vi "EngineTagsUI.vi"() -> ()   [LabVIEW 2013, in "PL Framework Configuration Tool.lvlib" / "Engine Mappings.lvclass"]
uses:
  Engine Mappings.lvclass
  <vilib>/CEF_TreeControl/Node/NodeRef.ctl
  <vilib>/CEF_TreeControl/Node/NISE_CEF_Node.lvclass
  <vilib>/NI/AMC/Message Queue.ctl
  <vilib>/NI/AMC/Message.ctl
  <vilib>/NI/Tools/Keyed Array/KeyedArray.ctl
  <vilib>/CEF_TreeControl/Node/UserEventRef.ctl
  <vilib>/CEF_TreeControl/Controls/EventCluster.ctl
  <vilib>/NI/Tag Bus Module Framework/root configuration/TBM configuration.lvclass/TBM configuration.ctl
  <vilib>/NI/Tag Bus/tag/tag descriptor.lvclass/tag descriptor.ctl
  Engine Parent/read engine configuration.vi
  <vilib>/NI/Tag Bus Module Framework/root configuration/create GUID.vi
  Engine Parent/write engine configuration.vi
  <vilib>/NI/Module Execution Interface/Engine Configuration/engine configuration.lvclass
  <vilib>/NI/Tag Bus Module Framework/root configuration/TBM configuration.lvclass
  Engine Parent/Engine Parent Editor Node.lvclass
  <vilib>/CEF_TreeControl/NISE_CEF_TreeControl.lvlib
  <vilib>/NI/Tag Bus/tag/tag descriptor.lvclass
  <vilib>/NI/Tools/Keyed Array/Tools_KeyedArray.lvlib
  <vilib>/NI/AMC/AMC.lvlib
panel:
  in  "channels":i32(listbox)
  in  "main queue":T1
  in  "node ref":T2
  in  "Tags":i32(listbox)
  in  "user event":T3
  in  "unmap":bool
  in  "map":bool
  in  "Mappings":i32(listbox)
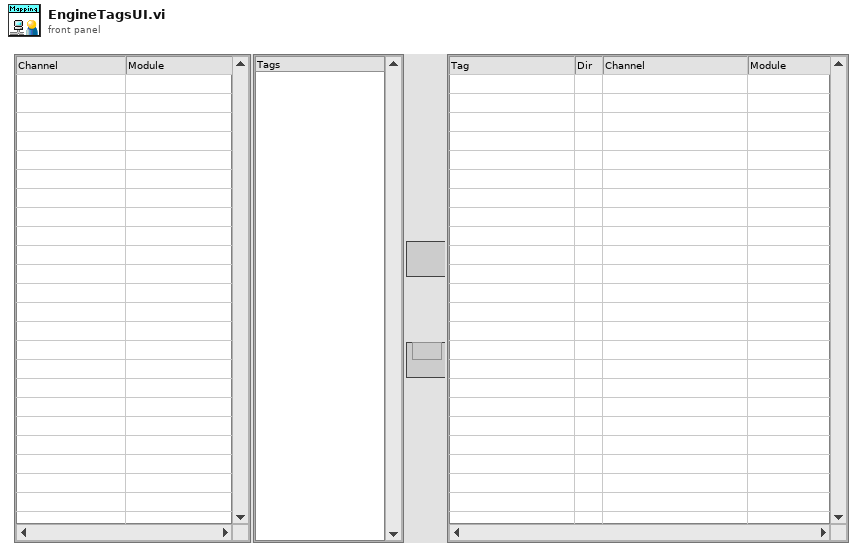
[diagram p1: front panel]
types:
  T1 = typedef "AMC.lvlib/Message Queue.ctl" = refnum<queue>
  T2 = typedef "NISE_CEF_Node.lvclass/NodeRef.ctl" = refnum<data-value>
  T3 = typedef "NISE_CEF_Node.lvclass/UserEventRef.ctl" = refnum<user-event>
  T4 = typedef "NISE_CEF_TreeControl.lvlib/EventCluster.ctl" = cluster{"command":string, "data":string}
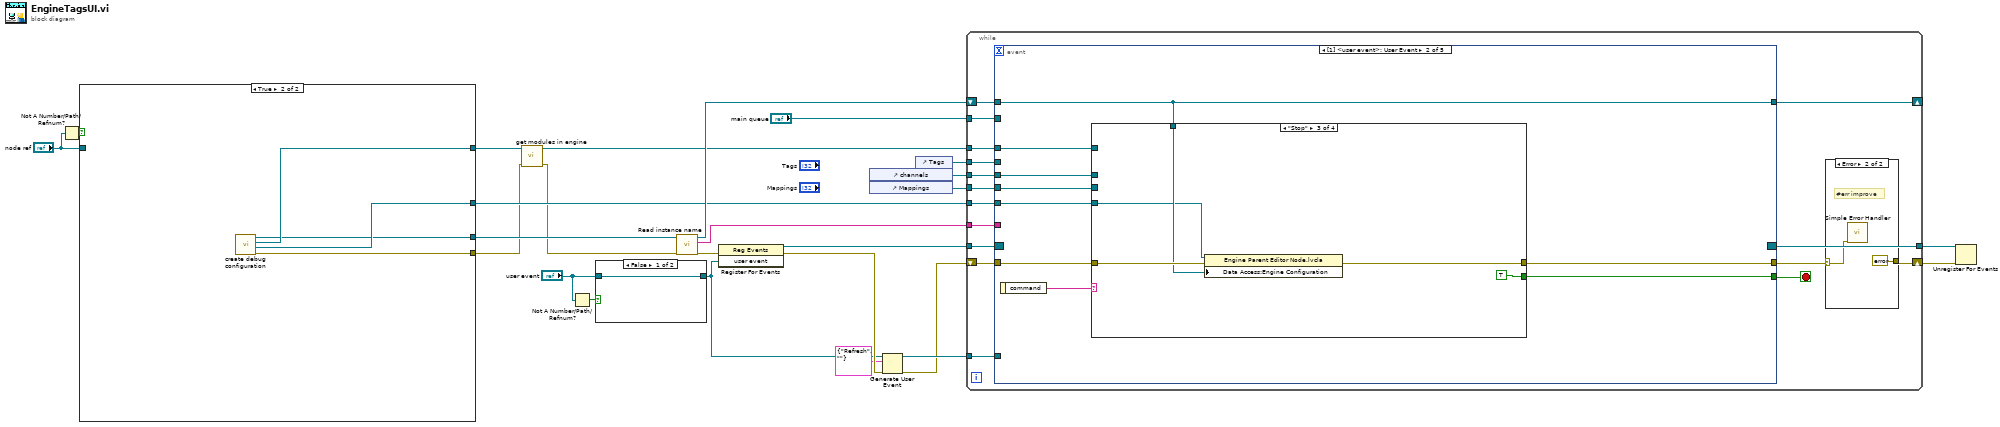
[diagram p0: block diagram]
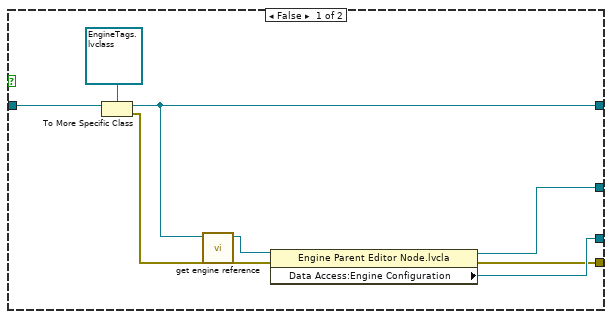
[diagram p2: hidden frame]
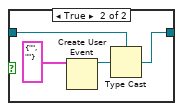
[diagram p3: hidden frame]
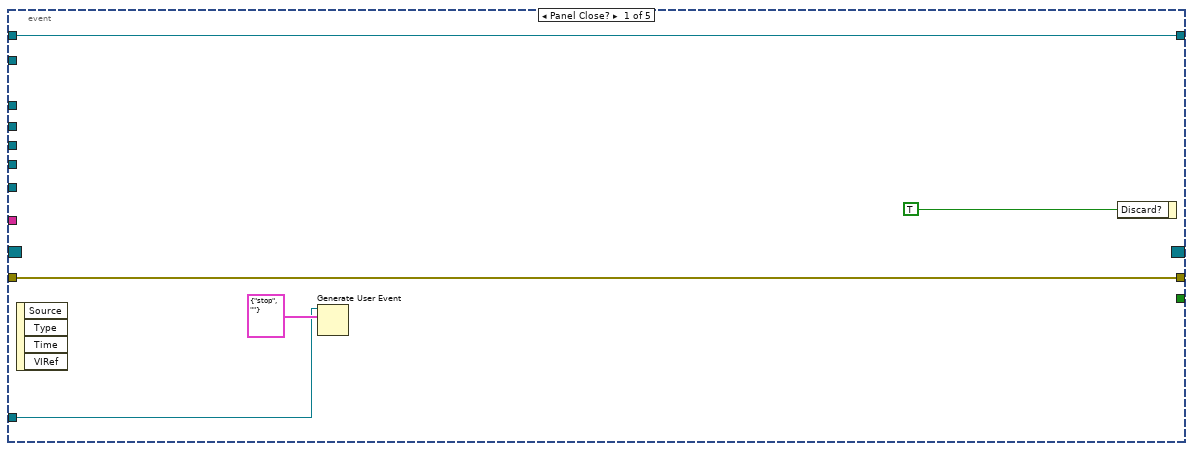
[diagram p5: hidden frame]
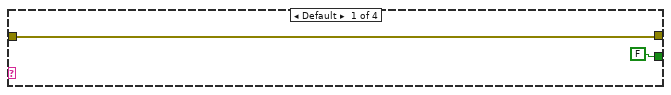
[diagram p6: hidden frame]
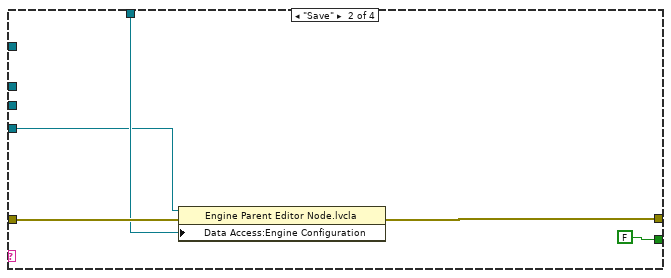
[diagram p7: hidden frame]
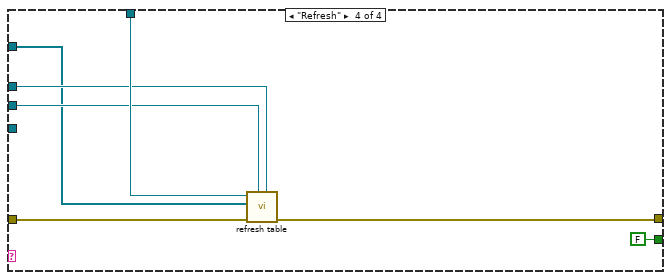
[diagram p8: hidden frame]
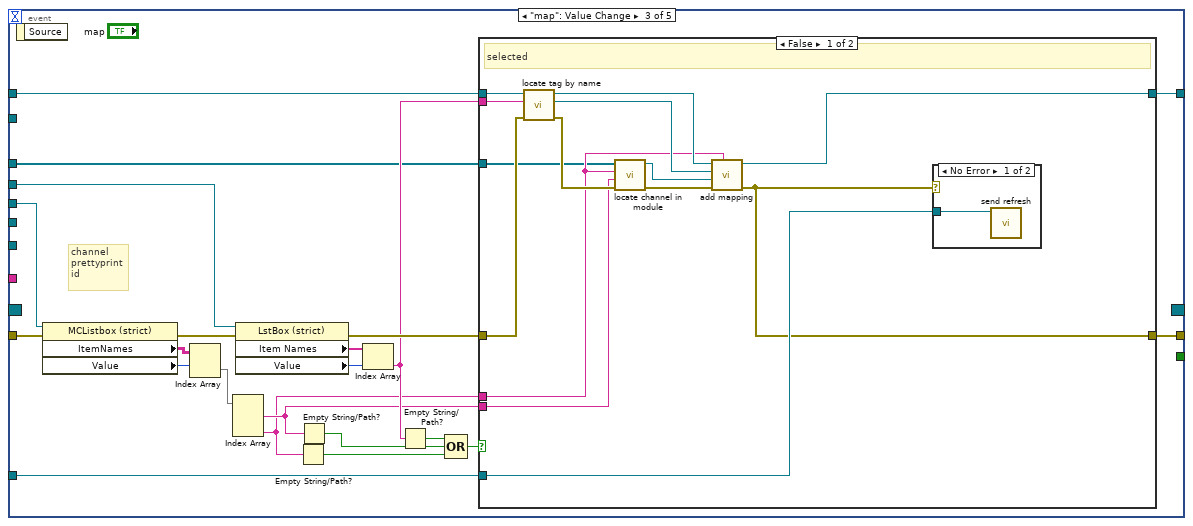
[diagram p9: hidden frame]
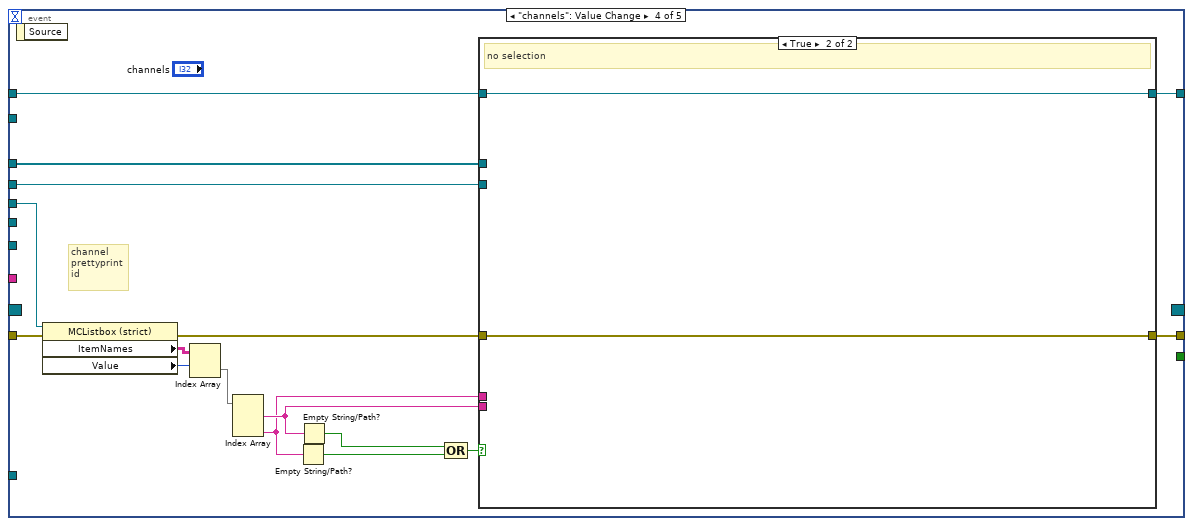
[diagram p12: hidden frame]
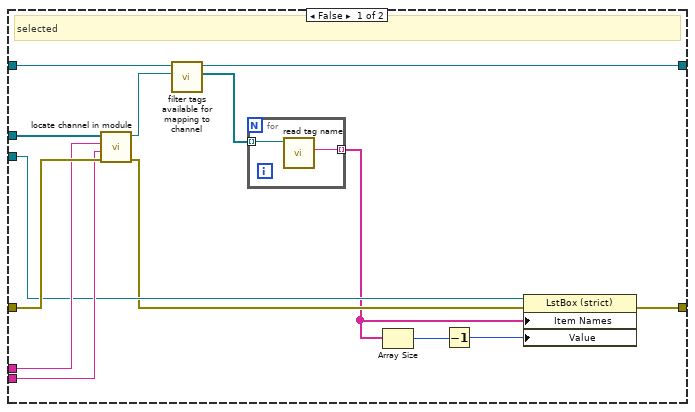
[diagram p13: hidden frame]
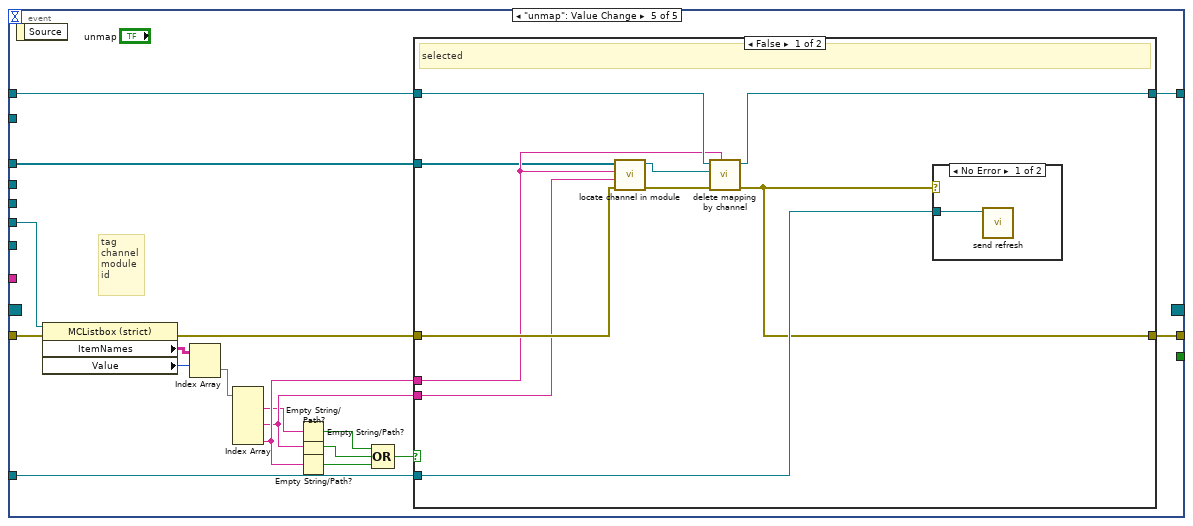
[diagram p14: hidden frame]
diagram:
  n1 = Not A Number/Path/Refnum?(number/path/refnum="node ref") -> (NaN/Path/Refnum?=w12:bool)
  n2 = case shown="True" w12 {
    tunnel: [w31 w37] -> w4
    tunnel: [w29 w36] -> w19
    tunnel: [w28 w35] -> w2
    tunnel: [w27 w38] -> w16
    tunnel: "node ref" -> [w26 _]
    frame False {
      n3 = To More Specific Class(target class=refnum<data-value> refnum ("data value reference"), reference=w26) -> (specific class reference=w31:refnum<data-value>, error out=w33:errorcluster)  [unwired: 1 in]
      n4 = call "get engine reference.vi"("error in"=w33, "engine mappings"=w31) -> ("error out"=w32:errorcluster, "engine reference"=w30:refnum<data-value>)  [unwired: 8 in]
      n5 = property class="Engine Parent Editor Node.lvcla"(reference=w30, error in=w32) -> (reference out=w27:refnum<data-value>, error out=w28:errorcluster, "Data Access:Engine Configuration"=w29:refnum<class "engine configuration.lvclass">)
    }
    frame True {
      n6 = call "create debug configuration.vi"() -> ("error out"=w35:errorcluster, "engine dvr"=w38:refnum<data-value>, "mapping dvr"=w37:refnum<data-value>, "engine configuration out"=w36:refnum<class "engine configuration.lvclass">)  [unwired: 8 in]
    }
  }
  n7 = call "get modules in engine.vi"("error in"=w2, "engine mapping"=w4) -> ("error out"=w1:errorcluster, "Modules Configurations"=w3:refnum<class "TBM module configuration.lvclass">[])  [unwired: 8 in]
  n8 = Not A Number/Path/Refnum?(number/path/refnum="user event") -> (NaN/Path/Refnum?=w14:bool)
  n9 = case shown="False" w14 {
    tunnel: [w39 w40] -> w11
    tunnel: "user event" -> [w39 w41]
    frame False {
    }
    frame True {
      n10 = Create User Event(user event datatype=T4 {"command"="", "data"=""} ("event data")) -> (user event=w42:refnum<user-event>)  [unwired: 1 in, 1 out]
      n11 = Type Cast(type=w41, x=w42) -> (*(type *) &x=w40:T3)
    }
  }
  n12 = call <vilib>:"Read instance name.vi"("error in"=w1, "configuration in"=w19) -> ("error out"=w17:errorcluster, "instance id"=w18:string, "configuration out"=w20:refnum<class "engine configuration.lvclass">)  [unwired: 7 in]
  n13 = register-events(error in=w17, w11) -> (reference out=w24:refnum<event-registration>, error out=w21:errorcluster)  [unwired: 1 in]
  n14 = control-ref of="channels"() -> (w6:refnum<vi>)
  n15 = control-ref of="Mappings"() -> (w5:refnum<vi>)
  n16 = Generate User Event(user event=w11, event data cluster=T4 {"command"="Refresh", "data"=""} ("event data"), error in=w21) -> (user event out=w10:T3, error out=w9:errorcluster)  [unwired: 1 in]
  n17 = control-ref of="Tags"() -> (w7:refnum<vi>)
  n18 = while {
    tunnel: "main queue" -> [w59]
    tunnel: w24 -> [w58]
    tunnel: [w57] -> w23
    shift-right: [w55] -> _
    shift-left: w20 -> [w50]
    shift-right: [w54] -> w22
    shift-left: w9 -> [w53]
    tunnel: w18 -> [w52]
    tunnel: w16 -> [w51]
    tunnel: w10 -> [w48]
    tunnel: w7 -> [w47]
    tunnel: w6 -> [w46]
    tunnel: w5 -> [w45]
    tunnel: w3 -> [w44]
    stop <- w56 stop-if-true
    n19 = event shown="[1] <user event>: User Event" {
      selector: w58 -> [_ _ _ _ _]
      dyn-events: [_ _ _ _ _] -> w57
      timeout: _ -> [_ _ _ _ _]
      tunnel: w59 -> [_ _ _ _ _]
      tunnel: [_ w72 _ _ _] -> w56
      tunnel: w50 -> [w67 w74 w103 w140 w178]
      tunnel: [w67 w74 w104 w141 w179] -> w55
      tunnel: w53 -> [w66 w76 w117 w150 w186]
      tunnel: [w66 w75 w101 w139 w177] -> w49
      tunnel: w52 -> [_ _ _ _ _]
      tunnel: w51 -> [_ w73 _ _ _]
      tunnel: w48 -> [w64 _ w100 _ w176]
      tunnel: w47 -> [_ _ w116 w135 _]
      tunnel: w46 -> [_ w70 w114 w148 _]
      tunnel: w45 -> [_ w69 _ _ w175]
      tunnel: w44 -> [_ w68 w96 w136 w169]
      event Panel Close? {
        n20 = event-data() -> ()  [unwired: 1 in, 4 out]
        n21 = Generate User Event(user event=w64, event data cluster=T4 {"command"="stop", "data"=""} ("event data")) -> ()  [unwired: 2 in, 2 out]
        n22 = event-data("Discard?"=TRUE) -> ()  [unwired: 1 in, 1 out]
      }
      event User Event {
        n23 = event-data() -> ("command"=w71:string)  [unwired: 1 in]
        n24 = case shown="\"Stop\"" w71 {
          tunnel: w76 -> [w78 w83 w88 w93]
          tunnel: [w78 w82 w87 w92] -> w75
          tunnel: w74 -> [_ w81 w86 w94]
          tunnel: w73 -> [_ w80 w85 _]
          tunnel: [FALSE FALSE TRUE FALSE] -> w72
          tunnel: w70 -> [_ _ _ w91]
          tunnel: w69 -> [_ _ _ w90]
          tunnel: w68 -> [_ _ _ w89]
          frame Default {
          }
          frame "Save" {
            n25 = property class="Engine Parent Editor Node.lvcla"(reference=w80, error in=w83, "Data Access:Engine Configuration"=w81) -> (error out=w82:errorcluster)  [unwired: 1 out]
          }
          frame "Stop" {
            n26 = property class="Engine Parent Editor Node.lvcla"(reference=w85, error in=w88, "Data Access:Engine Configuration"=w86) -> (error out=w87:errorcluster)  [unwired: 1 out]
          }
          frame "Refresh" {
            n27 = call "refresh table.vi"("channels ref"=w91, "Mappings"=w90, "error in"=w93, "Modules Configurations"=w89, "engine configuration in"=w94) -> ("error out"=w92:errorcluster)  [unwired: 6 in]
          }
        }
      }
      event "map": Value Change {
        # "channel\nprettyprint\nid"
        n28 = event-data() -> ()  [unwired: 1 in, 1 out]
        n29 = property class="MCListbox (strict)"(reference=w114, error in=w117) -> (error out=w115:errorcluster, "ItemNames"=w112:string[][], "Value"=w113:i32)  [unwired: 1 out]
        n30 = Index Array(array=w112, index (row)=w113) -> (element=w109:string[])  [unwired: 1 in]
        n31 = Index Array(array=w109) -> (element #1=w98:string, element #3=w97:string)  [unwired: 3 in, 1 out]
        n32 = property class="LstBox (strict)"(reference=w116, error in=w115) -> (error out=w102:errorcluster, "Item Names"=w111:string[], "Value"=w110:i32)  [unwired: 1 out]
        n33 = Empty String/Path?(string/path=w97) -> (empty?=w108:bool)
        n34 = Empty String/Path?(string/path=w98) -> (empty?=w107:bool)
        n35 = Index Array(array=w111, index=w110) -> (element=w99:string)
        n36 = Empty String/Path?(string/path=w99) -> (empty?=w106:bool)
        n37 = Compound Arithmetic op=OR(w106, w107, w108) -> (w105:bool)
        n38 = case shown="False" w105 {
          tunnel: [w124 w134] -> w104
          tunnel: w103 -> [w130 w134]
          tunnel: w102 -> [w129 w133]
          tunnel: [w119 w133] -> w101
          tunnel: w100 -> [w131 _]
          tunnel: w99 -> [w128 _]
          tunnel: w98 -> [w126 _]
          tunnel: w97 -> [w120 _]
          tunnel: w96 -> [w118 _]
          frame False {
            # "selected"
            n39 = call <vilib>:"locate tag by name.vi"("error in"=w129, "tag name"=w128, "engine configuration in"=w130) -> ("error out"=w127:errorcluster, "tag descriptor"=w122:refnum<class "tag descriptor.lvclass">, "engine configuration out"=w125:refnum<class "engine configuration.lvclass">)  [unwired: 6 in]
            n40 = call "locate channel in module.vi"("error in"=w127, "channel name"=w126, "instance id"=w120, "Modules Configurations"=w118) -> ("error out"=w123:errorcluster, "channel"=w121:refnum<class "TBM channel.lvclass">)  [unwired: 6 in]
            n41 = call <vilib>:"add mapping.vi"("owner ID"=w120, "error in"=w123, "channel"=w121, "tag descriptor"=w122, "engine configuration"=w125) -> ("error out"=w119:errorcluster, "engine configuration out"=w124:refnum<class "engine configuration.lvclass">)  [unwired: 5 in]
            n42 = case shown="No Error" w119 {
              tunnel: w131 -> [w132 _]
              frame No Error {
                n43 = call "send refresh.vi"("User Event in"=w132) -> ()  [unwired: 11 in]
              }
              frame Error {
              }
            }
          }
          frame True {
            # "no selection"
          }
        }
      }
      event "channels": Value Change {
        # "channel\nprettyprint\nid"
        n44 = event-data() -> ()  [unwired: 1 in, 1 out]
        n45 = property class="MCListbox (strict)"(reference=w148, error in=w150) -> (error out=w149:errorcluster, "ItemNames"=w146:string[][], "Value"=w147:i32)  [unwired: 1 out]
        n46 = Index Array(array=w146, index (row)=w147) -> (element=w145:string[])  [unwired: 1 in]
        n47 = Index Array(array=w145) -> (element #1=w138:string, element #3=w137:string)  [unwired: 3 in, 1 out]
        n48 = Empty String/Path?(string/path=w137) -> (empty?=w144:bool)
        n49 = Empty String/Path?(string/path=w138) -> (empty?=w143:bool)
        n50 = Compound Arithmetic op=OR(w143, w144) -> (w142:bool)
        n51 = case shown="True" w142 {
          tunnel: [w154 w168] -> w141
          tunnel: w140 -> [w160 w168]
          tunnel: w149 -> [w164 w167]
          tunnel: [w157 w167] -> w139
          tunnel: w138 -> [w163 _]
          tunnel: w137 -> [w162 _]
          tunnel: w136 -> [w161 _]
          tunnel: w135 -> [w158 _]
          frame False {
            # "selected"
            n52 = call "locate channel in module.vi"("error in"=w164, "channel name"=w163, "instance id"=w162, "Modules Configurations"=w161) -> ("error out"=w156:errorcluster, "channel"=w159:refnum<class "TBM channel.lvclass">)  [unwired: 6 in]
            n53 = call <vilib>:"filter tags available for mapping to channel.vi"("channel to map to"=w159, "engine configuration in"=w160) -> ("filtered tags"=w155:refnum<class "tag descriptor.lvclass">[], "engine configuration out"=w154:refnum<class "engine configuration.lvclass">)  [unwired: 8 in]
            n54 = for {
              tunnel: w155 -> [w166] mode=indexing
              tunnel: [w165] -> w153 mode=indexing
              n55 = call <vilib>:"read tag name.vi"("system tag in"=w166) -> ("name"=w165:string)  [unwired: 8 in, 2 out]
            }
            n56 = Array Size(array=w153) -> (size(s)=w152:i32)
            n57 = Decrement(x=w152) -> (x-1=w151:i32)
            n58 = property class="LstBox (strict)"(reference=w158, error in=w156, "Item Names"=w153, "Value"=w151) -> (error out=w157:errorcluster)  [unwired: 1 out]
          }
          frame True {
            # "no selection"
          }
        }
      }
      event "unmap": Value Change {
        # "tag\nchannel\nmodule\nid"
        n59 = event-data() -> ()  [unwired: 1 in, 1 out]
        n60 = property class="MCListbox (strict)"(reference=w175, error in=w186) -> (error out=w185:errorcluster, "ItemNames"=w183:string[][], "Value"=w184:i32)  [unwired: 1 out]
        n61 = Index Array(array=w183, index (row)=w184) -> (element=w182:string[])  [unwired: 1 in]
        n62 = Index Array(array=w182) -> (element #1=w170:string, element #3=w171:string, element #5=w174:string)  [unwired: 5 in, 2 out]
        n63 = Empty String/Path?(string/path=w170) -> (empty?=w172:bool)
        n64 = Empty String/Path?(string/path=w171) -> (empty?=w173:bool)
        n65 = Empty String/Path?(string/path=w174) -> (empty?=w181:bool)
        n66 = Compound Arithmetic op=OR(w172, w173, w181) -> (w180:bool)
        n67 = case shown="False" w180 {
          tunnel: [w190 w199] -> w179
          tunnel: w178 -> [w191 w199]
          tunnel: w185 -> [w195 w198]
          tunnel: [w188 w198] -> w177
          tunnel: w176 -> [w196 _]
          tunnel: w171 -> [w194 _]
          tunnel: w174 -> [w189 _]
          tunnel: w169 -> [w187 _]
          frame False {
            # "selected"
            n68 = call "locate channel in module.vi"("error in"=w195, "channel name"=w194, "instance id"=w189, "Modules Configurations"=w187) -> ("error out"=w193:errorcluster, "channel"=w192:refnum<class "TBM channel.lvclass">)  [unwired: 6 in]
            n69 = call <vilib>:"delete mapping by channel.vi"("owner ID"=w189, "error in"=w193, "channel"=w192, "engine configuration in"=w191) -> ("error out"=w188:errorcluster, "engine configuration out"=w190:refnum<class "engine configuration.lvclass">)  [unwired: 6 in]
            n70 = case shown="No Error" w188 {
              tunnel: w196 -> [w197 _]
              frame No Error {
                n71 = call "send refresh.vi"("User Event in"=w197) -> ()  [unwired: 11 in]
              }
              frame Error {
              }
            }
          }
          frame True {
            # "no selection"
          }
        }
      }
    }
    n72 = case shown="Error" w49 {
      selector: w49 -> [w60 w62]
      tunnel: [w60 errorcluster {"status"=FALSE, "code"=0, "source"=""} ("error IO")] -> w54
      frame No Error {
      }
      frame Error {
        # "#err improve"
        n73 = call <vilib>:"Simple Error Handler.vi"("error in (no error)"=w62) -> ()  [unwired: 4 in, 5 out]
      }
    }
  }
  n74 = Unregister For Events(event registration refnum=w23, error in=w22) -> ()  [unwired: 1 out]
